vi "Register DoubleClick Callback.vi"(8 "error in":errorcluster, 10 "onDoubleClick":refnum<user-event>, 11 "Custom Events in":refnum<class "Custom Events.lvclass">) -> (0 "error out":errorcluster, 2 "Event Callback Refnum":refnum<k27>, 3 "Custom Events out":refnum<class "Custom Events.lvclass">)   [LabVIEW 2023, in "SourceGrid.lvlib" / "Custom Events.lvclass"]
uses:
  Custom Events.lvclass
  Cells/Cell Context/Cell Context.lvclass
  DoubleClick Callback.vi
  D:/git/Sourcegrid-LabVIEW/dll/SourceGrid.dll
  dll/SourceGrid.dll
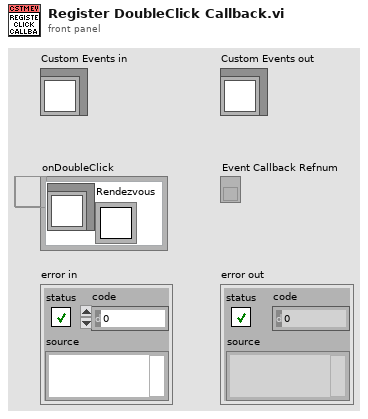
[diagram p1: front panel]
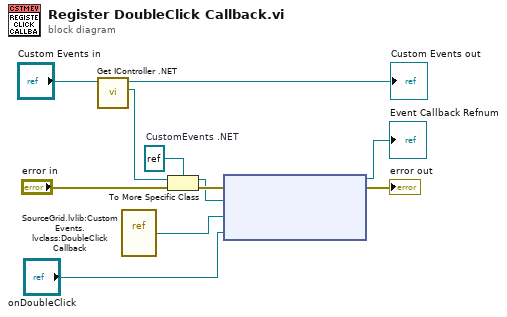
[diagram p0: block diagram]
diagram:
  w1 = refnum<k24> refnum  # CustomEvents .NET
  n1 = call-dynamic "Get IController .NET.vi"("Custom Events in"="Custom Events in") -> ("IController"=w2:refnum<k24>, "Custom Events out"=→"Custom Events out":refnum<class "Custom Events.lvclass">)  [unwired: 9 in]
  n2 = vi-ref "SourceGrid.lvlib:Custom Events.lvclass:DoubleClick Callback.vi"() -> (w5:refnum<vi>)
  n3 = To More Specific Class(target class=w1, reference=w2, error in="error in") -> (specific class reference=w3:refnum<k24>, error out=w4:errorcluster)
  n4 = node(w4, w3, w5, "onDoubleClick") -> (→"Event Callback Refnum":refnum<k27>, →"error out":errorcluster)  [unwired: 1 in]
